vi "PicoScope4000GetRapidBlock.vi"(0 "error in":errorcluster, 7 "handle in":i16, 11 "Rapid Block Acquisition Settings":T1) -> (2 "Channel A Buffer":i16[][](array[numeric]), 3 "Channel B Buffer":i16[][](array[numeric]), 4 "error out":errorcluster, 6 "handle out":i16, 13 "Channel C Buffer":i16[][](array[numeric]), 14 "Channel D Buffer":i16[][](array[numeric]))   [LabVIEW 2009]
doc: "This VI gets a set of blocks captured using rapid block mode. It outputs two-dimensional arrays for each channel that contain data from all the requested captures."
uses:
  Program Files/Pico Technology/SDK/lib/ps4000.dll
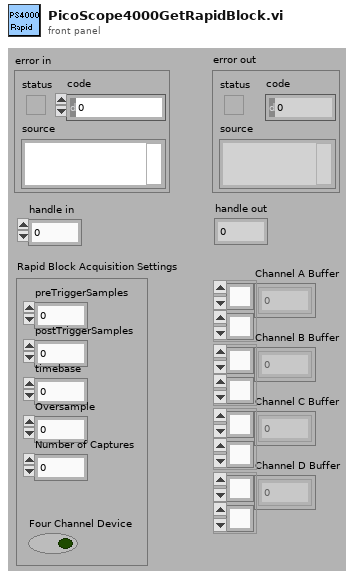
[diagram p1: front panel]
types:
  T1 = cluster{"preTriggerSamples":i32, "postTriggerSamples":i32, "timebase":u32, "Four Channel Device":bool, "Oversample":i16, "Number of Captures":i16}
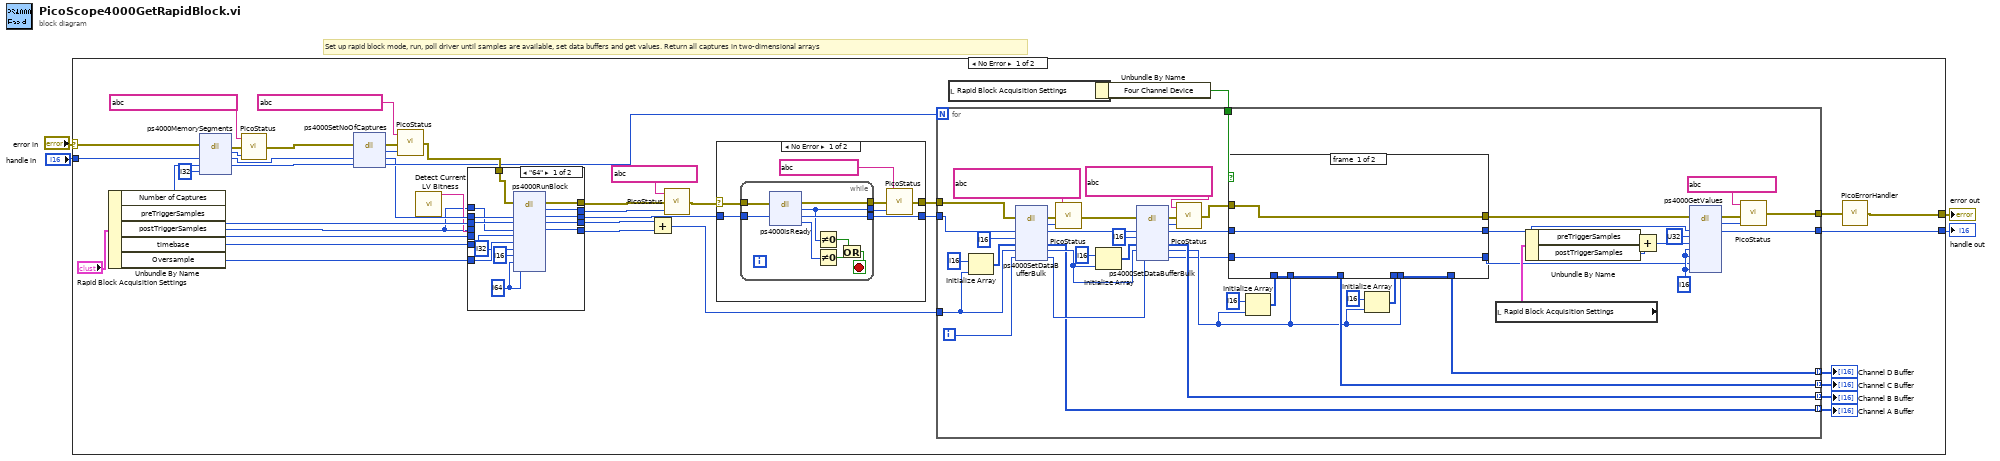
[diagram p0: block diagram]
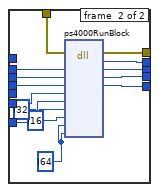
[diagram p2: hidden frame]
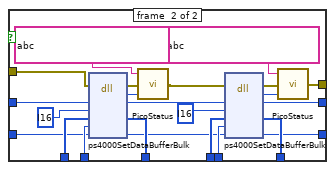
[diagram p3: hidden frame]
diagram:
  # "Set up rapid block mode, run, poll driver until samples are available, set data buffers and get values. Return all captures in two-dimensional arrays"
  n1 = case shown="No Error" "error in" {
    selector: "error in" -> [w33 w168]
    tunnel: [w9 w168] -> w3
    tunnel: "handle in" -> [w32 w167]
    tunnel: [w11 w167] -> w1
    frame #0 {
      n2 = Unbundle By Name("Rapid Block Acquisition Settings") -> ("Number of Captures"=w28:i16, "preTriggerSamples"=w39:i32, "postTriggerSamples"=w7:i32, "timebase"=w5:u32, "Oversample"=w6:i16)
      n3 = dll-call lib="C:/Program Files/Pico Technology/SDK/lib/PS4000.dll" fn="ps4000MemorySegments" ("ps3000.dll:_ps3000_open_unit@0")(error in=w33, "handle"=w32, "nSegments"=w28, "nMaxSamples"=i32 ?) -> (error out=w30:errorcluster, "PICO_STATUS"=w31:i32, "handle"=w25:i16, "nSegments"=w26:u16)  [unwired: 3 in, 1 out]
      n4 = call "PicoStatus.vi"("PICO STATUS"=w31, "error in"=w30, "source"=string ?) -> ("error out"=w24:errorcluster)
      n5 = dll-call lib="C:/Program Files/Pico Technology/SDK/lib/PS4000.dll" fn="ps4000SetNoOfCaptures" ("ps3000.dll:_ps3000_open_unit@0")(error in=w24, "handle"=w25, "nCaptures"=w26) -> (error out=w22:errorcluster, "PICO_STATUS"=w23:i32, "handle"=w16:i16, "nCaptures"=w17:u16)  [unwired: 2 in, 1 out]
      n6 = call "PicoStatus.vi"("PICO STATUS"=w23, "error in"=w22, "source"=string ?) -> ("error out"=w20:errorcluster)
      n7 = call "Detect Current LV Bitness.vi"() -> ("bitness"=w8:string)  [unwired: 11 in]
      n8 = case shown="\"64\"" w8 {
        tunnel: [w51 w73] -> w45
        tunnel: [w50 w72] -> w43
        tunnel: [w49 w71] -> w42
        tunnel: w5 -> [_ _]
        tunnel: w39 -> [w57 w70]
        tunnel: w7 -> [_ w69]
        tunnel: [w52 w68] -> w37
        tunnel: [w53 w67] -> w36
        tunnel: w20 -> [w59 w66]
        tunnel: w16 -> [w58 w65]
        tunnel: w7 -> [w56 _]
        tunnel: w6 -> [w55 w64]
        tunnel: w5 -> [w54 w63]
        frame #0 {
          w46 = i64 ? ("pParameter")
          n9 = dll-call lib="C:/Program Files/Pico Technology/SDK/lib/ps4000.dll" fn="ps4000RunBlock" ("ps3000.dll:_ps3000_open_unit@0")(error in=w59, "handle"=w58, "preTriggerSamples"=w57, "postTriggerSamples"=w56, "timebase"=w54, "oversample"=w55, "timeindisposed"=i32 ?, "segmentIndex"=i16 ?, "lpReady"=w46, "pParameter"=w46) -> (error out=w53:errorcluster, "PICO_STATUS"=w52:i32, "handle"=w51:i16, "preTriggerSamples"=w50:i32, "postTriggerSamples"=w49:i32)  [unwired: 8 in, 1 out]
        }
        frame #1 {
          w60 = i64 ? ("pParameter")
          n10 = dll-call lib="C:/Program Files/Pico Technology/SDK/lib/PS4000.dll" fn="ps4000RunBlock" ("ps3000.dll:_ps3000_open_unit@0")(error in=w66, "handle"=w65, "preTriggerSamples"=w70, "postTriggerSamples"=w69, "timebase"=w63, "oversample"=w64, "timeindisposed"=i32 ?, "segmentIndex"=i16 ?, "lpReady"=w60, "pParameter"=w60) -> (error out=w67:errorcluster, "PICO_STATUS"=w68:i32, "handle"=w73:i16, "preTriggerSamples"=w72:i32, "postTriggerSamples"=w71:i32)  [unwired: 8 in, 1 out]
        }
      }
      n11 = Add(x=w43, y=w42) -> (x+y=w19:i32)
      n12 = call "PicoStatus.vi"("PICO STATUS"=w37, "error in"=w36, "source"=string ?) -> ("error out"=w35:errorcluster)
      n13 = case shown="No Error" w35 {
        selector: w35 -> [w153 w165]
        tunnel: w45 -> [w155 w166]
        tunnel: [w154 w166] -> w44
        tunnel: [w152 w165] -> w41
        frame #0 {
          n14 = while {
            tunnel: [w164] -> w154
            tunnel: w155 -> [w163]
            tunnel: [w158] -> w150
            tunnel: w153 -> [w157]
            tunnel: [w156] -> w151
            stop <- w162 stop-if-true
            n15 = dll-call lib="C:/Program Files/Pico Technology/SDK/lib/ps4000.dll" fn="ps4000IsReady" ("ps3000.dll:_ps3000_open_unit@0")(error in=w157, "handle"=w163) -> (error out=w156:errorcluster, "status"=w158:i32, "handle"=w164:i16, "ready"=w159:i16)  [unwired: 3 in, 1 out]
            n16 = Not Equal To 0?(x=w158) -> (x != 0?=w160:bool)
            n17 = Not Equal To 0?(x=w159) -> (x != 0?=w161:bool)
            n18 = Or(x=w160, y=w161) -> (x .or. y?=w162:bool)
          }
          n19 = call "PicoStatus.vi"("PICO STATUS"=w150, "error in"=w151, "source"=string ?) -> ("error out"=w152:errorcluster)
        }
        frame #1 {
        }
      }
      n20 = local read "Rapid Block Acquisition Settings"() -> (w18:T1)
      n21 = Unbundle By Name(w18) -> ("Four Channel Device"=w38:bool)
      n22 = for {
        N: w17 -> [_]
        tunnel: w44 -> [w120]
        tunnel: w41 -> [w110]
        tunnel: w38 -> [w94]
        tunnel: [w98] -> w15 mode=indexing
        tunnel: [w97] -> w14 mode=indexing
        tunnel: [w96] -> w13 mode=indexing
        tunnel: [w88] -> w12 mode=indexing
        tunnel: w19 -> [w95]
        tunnel: [w75] -> w11
        tunnel: [w74] -> w10
        i -> [w91]
        w87 = i16 ? ("overflow")
        n23 = Initialize Array(i16 ? ("element"), w95) -> (w117:i16[])
        n24 = dll-call lib="C:/Program Files/Pico Technology/SDK/lib/ps4000.dll" fn="ps4000SetDataBufferBulk" ("ps3000.dll:_ps3000_open_unit@0")(error in=w110, "handle"=w120, "channel"=i16 ?, "buffer"=w117, "bufferLth"=w95, "waveform"=w91) -> (error out=w107:errorcluster, "PICO_STATUS"=w108:i32, "handle"=w119:i16, "buffer"=w88:i16[], "bufferLth"=w93:i32, "waveform"=w90:u16)  [unwired: 3 in, 1 out]
        n25 = call "PicoStatus.vi"("PICO STATUS"=w108, "error in"=w107, "source"=string ?) -> ("error out"=w106:errorcluster)
        n26 = Initialize Array(i16 ? ("element"), w93) -> (w114:i16[])
        n27 = dll-call lib="C:/Program Files/Pico Technology/SDK/lib/PS4000.dll" fn="ps4000SetDataBufferBulk" ("ps3000.dll:_ps3000_open_unit@0")(error in=w106, "handle"=w119, "channel"=i16 ?, "buffer"=w114, "bufferLth"=w93, "waveform"=w90) -> (error out=w104:errorcluster, "PICO_STATUS"=w105:i32, "handle"=w118:i16, "buffer"=w96:i16[], "bufferLth"=w92:i32, "waveform"=w89:u16)  [unwired: 3 in, 1 out]
        n28 = call "PicoStatus.vi"("PICO STATUS"=w105, "error in"=w104, "source"=string ?) -> ("error out"=w103:errorcluster)
        n29 = Initialize Array(i16 ? ("element"), w92) -> (w113:i16[])
        n30 = Initialize Array(i16 ? ("element"), w92) -> (w112:i16[])
        n31 = case shown="True" w94 {
          tunnel: w118 -> [w123 w148]
          tunnel: [w123 w146] -> w77
          tunnel: w113 -> [w125 w145]
          tunnel: w112 -> [w124 w144]
          tunnel: [w124 w143] -> w98
          tunnel: [w125 w142] -> w97
          tunnel: w103 -> [w122 w139]
          tunnel: [w122 w133] -> w78
          tunnel: w92 -> [_ w130]
          tunnel: w92 -> [_ w129]
          tunnel: w89 -> [w121 w128]
          tunnel: [w121 w126] -> w76
          frame #0 {
          }
          frame #1 {
            n32 = dll-call lib="C:/Program Files/Pico Technology/SDK/lib/PS4000.dll" fn="ps4000SetDataBufferBulk" ("ps3000.dll:_ps3000_open_unit@0")(error in=w139, "handle"=w148, "channel"=i16 ?, "buffer"=w145, "bufferLth"=w130, "waveform"=w128) -> (error out=w137:errorcluster, "PICO_STATUS"=w138:i32, "handle"=w147:i16, "buffer"=w142:i16[], "waveform"=w127:u16)  [unwired: 4 in, 1 out]
            n33 = call "PicoStatus.vi"("PICO STATUS"=w138, "error in"=w137, "source"=string ?) -> ("error out"=w136:errorcluster)
            n34 = dll-call lib="C:/Program Files/Pico Technology/SDK/lib/PS4000.dll" fn="ps4000SetDataBufferBulk" ("ps3000.dll:_ps3000_open_unit@0")(error in=w136, "handle"=w147, "channel"=i16 ?, "buffer"=w144, "bufferLth"=w129, "waveform"=w127) -> (error out=w134:errorcluster, "PICO_STATUS"=w135:i32, "handle"=w146:i16, "buffer"=w143:i16[], "waveform"=w126:u16)  [unwired: 4 in, 1 out]
            n35 = call "PicoStatus.vi"("PICO STATUS"=w135, "error in"=w134, "source"=string ?) -> ("error out"=w133:errorcluster)
          }
        }
        n36 = local read "Rapid Block Acquisition Settings"() -> (w83:T1)
        n37 = Unbundle By Name(w83) -> ("preTriggerSamples"=w85:i32, "postTriggerSamples"=w84:i32)
        n38 = Add(x=w85, y=w84) -> (x+y=w86:i32)
        n39 = dll-call lib="C:/Program Files/Pico Technology/SDK/lib/PS4000.dll" fn="ps4000GetValues" ("ps3000.dll:_ps3000_open_unit@0")(error in=w78, "handle"=w77, "startIndex"=u32 ?, "noOfSamples"=w86, "downSampleRatio"=w87, "downSampleRatioMode"=w87, "segmentIndex"=w76, "overflow"=w87) -> (error out=w80:errorcluster, "PICO_STATUS"=w79:i32, "handle"=w75:i16)  [unwired: 8 in, 1 out]
        n40 = call "PicoStatus.vi"("PICO STATUS"=w79, "error in"=w80, "source"=string ?) -> ("error out"=w74:errorcluster)
      }
      "Channel D Buffer" <- w15
      "Channel C Buffer" <- w14
      "Channel B Buffer" <- w13
      "Channel A Buffer" <- w12
      n41 = call "PicoErrorHandler.vi"("error in"=w10) -> ("error out"=w9:errorcluster)
    }
    frame #1 {
    }
  }
  "error out" <- w3
  "handle out" <- w1
